vi "Close_Instr.vi"(8 "error in (no error)":errorcluster caption="entrée d'erreur (pas d'erreur)", 11 "Class Instrument Multimeter en entrée":refnum<class "Class Instrument LED_Analyser.lvclass">) -> (0 "error out":errorcluster caption="sortie d'erreur", 3 "Class Instrument Multimeter en sortie":refnum<class "Class Instrument LED_Analyser.lvclass">)   [LabVIEW 2020, in "Library Instrument & Equipement.lvlib" / "Library Instruments.lvlib" / "Class Instrument LED_Analyser.lvclass"]
uses:
  Class Instrument LED_Analyser.lvclass
  Class Instrument LED_Analyser.lvclass/Class Instrument LED_Analyser.ctl
  LED Analyser/Class Led Analyser (Default)/Class LED Analyser (Default).lvclass
  Instrument (Default)/Class Instrument (Default).lvclass
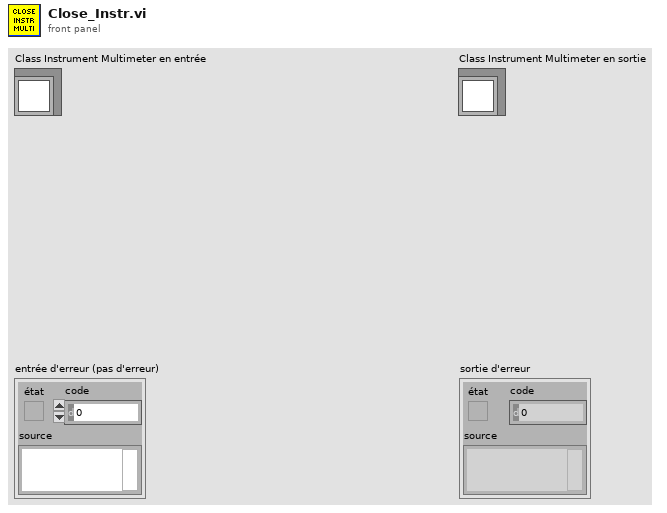
[diagram p1: front panel]
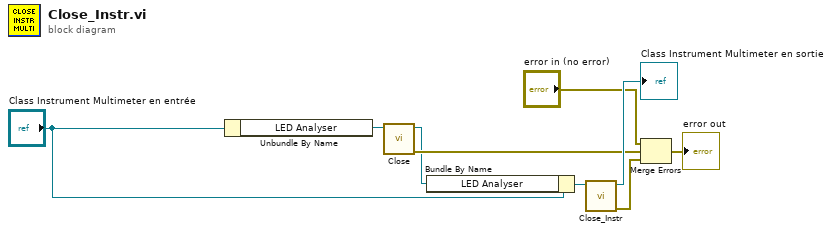
[diagram p0: block diagram]
diagram:
  n1 = Unbundle By Name("Class Instrument Multimeter en entrée") -> ("LED Analyser"=w3:refnum<class "Class LED Analyser (Default).lvclass">)
  n2 = call-dynamic "Close.vi"("Class LED Analyser in"=w3) -> ("error out"=w2:errorcluster, "Class LED Analyser Out"=w1:refnum<class "Class LED Analyser (Default).lvclass">)  [unwired: 9 in]
  n3 = Bundle By Name(cluster="Class Instrument Multimeter en entrée", "LED Analyser"=w1) -> (w7:refnum<class "Class Instrument LED_Analyser.lvclass">)
  n4 = call-parent "Close_Instr.vi"("Class Instrument (Default) en entrée"=w7) -> ("error out"=w5:errorcluster, "Class Instrument (Default) en sortie"=→"Class Instrument Multimeter en sortie":refnum<class "Class Instrument LED_Analyser.lvclass">)  [unwired: 9 in]
  n5 = Merge Errors("error in (no error)", w2, w5) -> (→"error out":errorcluster)
